vi "Actor Core.vi"(8 "error in":errorcluster, 11 "Task Setting Editor in":refnum<class "Task Setting Editor.lvclass">) -> (0 "error out":errorcluster, 3 "Actor out":refnum<class "Actor.lvclass">)   [LabVIEW 2017, in "Task Setting Editor.lvlib" / "Task Setting Editor.lvclass"]
doc: "(<B>Filename</B>: Actor Framework.lvlib:Actor.lvclass:Actor Core.vi)\n\nReceives messages to the actor, reacts to them, and initiates any error handling that may shut the actor down.\n\nDescendant classes may override this VI to append parallel tasks for the actor to complete while it handles messages. Overrides use the Call Parent Method node."
uses:
  Task Setting Editor.lvclass
  C:/Program Files (x86)/National Instruments/LabVIEW 2017/vi.lib/ActorFramework/Actor/Actor.lvclass
  C:/Users/Public/Documents/wc/BuildFarm/src/LabVIEW/vi.lib/BenjaminR/Build Farm/Actors/Framework/Actor wHelper/Actor wHelper.lvclass
  <vilib>/ActorFramework/Actor/Actor.lvclass
  Task Setting Editor.lvclass/Task Setting Editor.ctl
  <vilib>/ActorFramework/Actor/Actor.lvclass/Actor.ctl
  <vilib>/ActorFramework/Message Enqueuer/Message Enqueuer.lvclass/Message Enqueuer.ctl
  Framework/Actor wHelper/Actor wHelper.lvclass/Actor wHelper.ctl
  Task Setting Editor Messages/Update Task Infos Msg/Update Task Infos Msg.lvclass/Update Task Infos Msg.ctl
  Task Setting Editor Messages/Udpate Task Display Name Msg/Udpate Task Display Name Msg.lvclass/Udpate Task Display Name Msg.ctl
  Task Setting Editor Messages/Udpate Task Worker Msg/Udpate Task Worker Msg.lvclass/Udpate Task Worker Msg.ctl
  Task Setting Editor Messages/Send Task Settings Payload Msg/Send Task Settings Payload Msg.lvclass/Send Task Settings Payload Msg.ctl
  Framework/Actor wHelper/Read StopHelperLoop Reg Ref.vi
  <vilib>/ActorFramework/Message Enqueuer/Init from Existing Queue.vi
  <vilib>/ActorFramework/Message Enqueuer/Enqueue.vi
  Task Setting Editor Messages/Update Task Infos Msg/Update Task Infos Msg.lvclass
  C:/Program Files (x86)/National Instruments/LabVIEW 2017/vi.lib/ActorFramework/Message/Message.lvclass
  Task Setting Editor Messages/Udpate Task Display Name Msg/Udpate Task Display Name Msg.lvclass
  Task Setting Editor Messages/Udpate Task Worker Msg/Udpate Task Worker Msg.lvclass
  <vilib>/ActorFramework/Stop Msg/Stop Msg.lvclass
  Task Setting Editor Messages/Send Task Settings Payload Msg/Send Task Settings Payload Msg.lvclass
  <vilib>/ActorFramework/Message Priority Queue/Priority Enqueue.vi
  Framework/Actor wHelper/Actor wHelper.lvclass
  <vilib>/ActorFramework/Message Enqueuer/Message Enqueuer.lvclass
panel:
  in  "Task List":i32(listbox)
  out "Name":string
  in  "Worker":u16(ring)
  out "Status string":string
  out "BuildSpec Name":string
  out "BuildSpec Type":string
  out "Target":string
  out "ProjectPath":string
  out "ProjectName":string
  in  "Display Name":string
  in  "Cancel":bool
  in  "OK":bool
  out "modified?":bool
  # "Tasks"
  # "Infos"
  # "Worker"
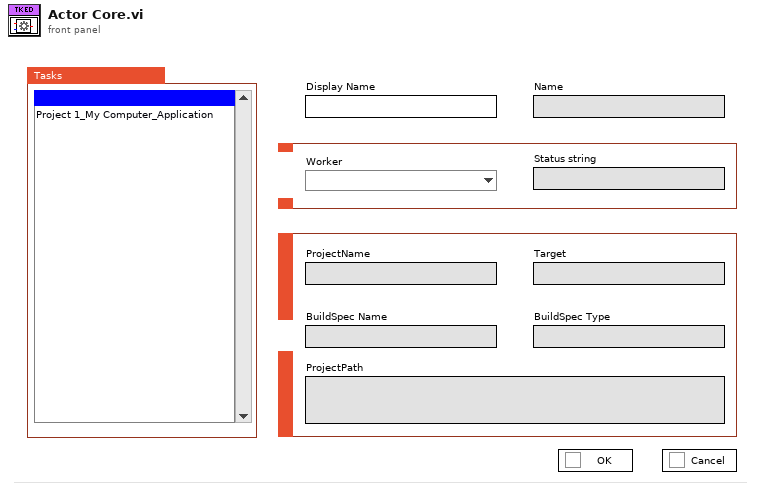
[diagram p1: front panel]
types:
  T1 = cluster{"Properties:StopHelperLoop Reg Ref":refnum<event-registration>}
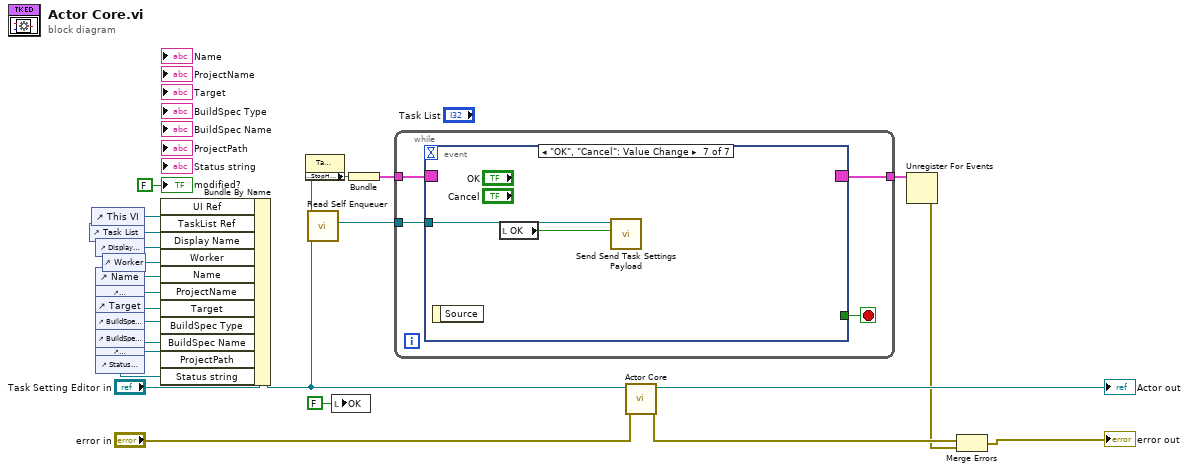
[diagram p0: block diagram]
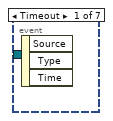
[diagram p2: hidden frame]
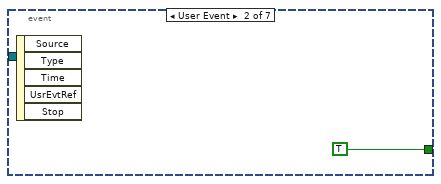
[diagram p3: hidden frame]
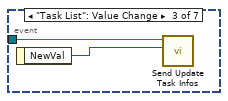
[diagram p4: hidden frame]
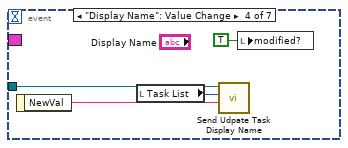
[diagram p5: hidden frame]
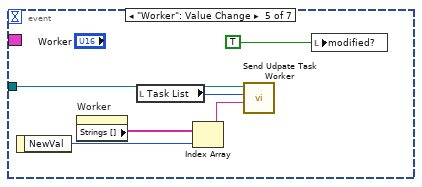
[diagram p6: hidden frame]
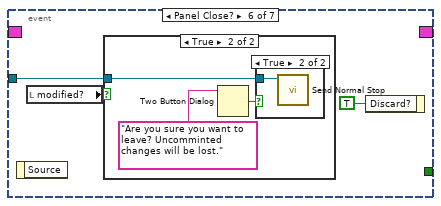
[diagram p7: hidden frame]
diagram:
  n1 = control-ref of="Task List"() -> (w17:refnum<vi>)
  n2 = control-ref of="This VI"() -> (w4:refnum<vi>)
  n3 = control-ref of="Display Name"() -> (w16:refnum<vi>)
  n4 = control-ref of="Name"() -> (w14:refnum<vi>)
  n5 = control-ref of="ProjectName"() -> (w13:refnum<vi>)
  n6 = control-ref of="Target"() -> (w12:refnum<vi>)
  n7 = control-ref of="BuildSpec Type"() -> (w11:refnum<vi>)
  n8 = control-ref of="BuildSpec Name"() -> (w10:refnum<vi>)
  n9 = control-ref of="ProjectPath"() -> (w9:refnum<vi>)
  n10 = control-ref of="Status string"() -> (w8:refnum<vi>)
  n11 = control-ref of="Worker"() -> (w15:refnum<vi>)
  n12 = Bundle By Name(cluster="Task Setting Editor in", "UI Ref"=w4, "TaskList Ref"=w17, "Display Name"=w16, "Worker"=w15, "Name"=w14, "ProjectName"=w13, "Target"=w12, "BuildSpec Type"=w11, "BuildSpec Name"=w10, "ProjectPath"=w9, "Status string"=w8) -> (w7:refnum<class "Task Setting Editor.lvclass">)
  n13 = property class="Task Setting Editor.lvclass"(reference=w7) -> ("Properties:StopHelperLoop Reg Ref"=w22:refnum<event-registration>)  [unwired: 1 in, 2 out]
  n14 = call <vilib>:"Read Self Enqueuer.vi"("Actor"=w7) -> ("Self Enqueuer"=w6:refnum<class "Message Enqueuer.lvclass">)  [unwired: 10 in]
  n15 = local write "OK"(FALSE ("OK")) -> ()
  n16 = Bundle("Properties:StopHelperLoop Reg Ref"=w22) -> (w20:T1)  [unwired: 1 in]
  n17 = while {
    tunnel: w20 -> [w28]
    tunnel: [w27] -> w19
    tunnel: w6 -> [w25]
    stop <- w26 stop-if-true
    n18 = event shown="[6] \"OK\", \"Cancel\": Value Change" {
      selector: w28 -> [_ _ _ _ _ _ _]
      dyn-events: [_ _ _ _ _ _ _] -> w27
      timeout: _ -> [_ _ _ _ _ _ _]
      tunnel: [_ TRUE _ _ _ _ _] -> w26
      tunnel: w25 -> [_ _ w31 w35 w41 w43 w50]
      event Timeout {
        n19 = event-data() -> ()  [unwired: 1 in, 3 out]
      }
      event User Event {
        n20 = event-data() -> ()  [unwired: 1 in, 5 out]
      }
      event "Task List": Value Change {
        n21 = event-data() -> ("NewVal"=w30:i32)  [unwired: 1 in]
        n22 = call "Send Update Task Infos.vi"("Task"=w30, "Message Enqueuer in"=w31) -> ()  [unwired: 8 in, 2 out]
      }
      event "Display Name": Value Change {
        n23 = event-data() -> ("NewVal"=w34:string)  [unwired: 1 in]
        n24 = local read "Task List"() -> (w33:i32)
        n25 = call "Send Udpate Task Display Name.vi"("Display Name"=w34, "Task"=w33, "Message Enqueuer in"=w35) -> ()  [unwired: 7 in, 2 out]
        n26 = local write "modified?"(TRUE ("modified?")) -> ()
      }
      event "Worker": Value Change {
        n27 = event-data() -> ("NewVal"=w38:u16)  [unwired: 1 in]
        n28 = property on="Worker" class="Ring (strict)"() -> ("Strings []"=w39:string[])  [unwired: 2 in, 2 out]
        n29 = local read "Task List"() -> (w40:i32)
        n30 = Index Array(array=w39, index=w38) -> (element=w37:string)
        n31 = call "Send Udpate Task Worker.vi"("Worker"=w37, "Task"=w40, "Message Enqueuer in"=w41) -> ()  [unwired: 7 in, 2 out]
        n32 = local write "modified?"(TRUE ("modified?")) -> ()
      }
      event Panel Close? {
        n33 = event-data() -> ()  [unwired: 1 in, 1 out]
        n34 = local read "modified?"() -> (w42:bool)
        n35 = case shown="True" w42 {
          tunnel: w43 -> [_ w47]
          frame False {
          }
          frame True {
            n36 = Two Button Dialog(message="Are you sure you want to leave? Uncomminted changes will be lost.") -> (T button?=w46:bool)  [unwired: 2 in]
            n37 = case shown="True" w46 {
              tunnel: w47 -> [_ w48]
              frame False {
              }
              frame True {
                n38 = call <vilib>:"Send Normal Stop.vi"("Message Enqueuer"=w48) -> ()  [unwired: 10 in, 1 out]
              }
            }
          }
        }
        n39 = event-data("Discard?"=TRUE) -> ()  [unwired: 1 in, 1 out]
      }
      event "OK", "Cancel": Value Change {
        n40 = event-data() -> ()  [unwired: 1 in, 1 out]
        n41 = local read "OK"() -> (w49:bool)
        n42 = call "Send Send Task Settings Payload.vi"("OK"=w49, "Message Enqueuer in"=w50) -> ()  [unwired: 8 in, 2 out]
      }
    }
  }
  n43 = call-parent "Actor Core.vi"("error in"="error in", "Actor in"=w7) -> ("error out"=w24:errorcluster, "Actor out"=→"Actor out":refnum<class "Actor.lvclass">)  [unwired: 8 in]
  n44 = Unregister For Events(event registration refnum=w19) -> (error out=w18:errorcluster)  [unwired: 1 in]
  n45 = Merge Errors(w24, w18) -> (→"error out":errorcluster)
  "modified?" <- FALSE ("modified?")
